vi "Authenticate without Token.vi"(5 "HTTP Method":T4, 6 "Body Parameters":T3[](array[typedef]), 7 "OAuth Credentials":T1={"Consumer Key"="", "Signature Method"=enum."HMAC-SHA1", "Token"="", "Version"="", "Token Secret"="", "Consumer Secret"=""}, 8 "error in (no error)":errorcluster, 9 "Header Parameters":T3[](array[typedef]), 10 "URL Parameters":T3[](array[typedef]), 11 "Base URL":string) -> (0 "error out":errorcluster, 1 "Header Value":string, 2 "Header Parameter":string, 3 "Full URL":string, 4 "Body":string)   [LabVIEW 2011, in "i3-oauth.lvlib"]
uses:
  i3-oauth.lvlib
  Controls/key-value-pairs.ctl
  Controls/HTTP Method.ctl
  Controls/OAuth Credentials.ctl
  Controls/Signature Method.ctl
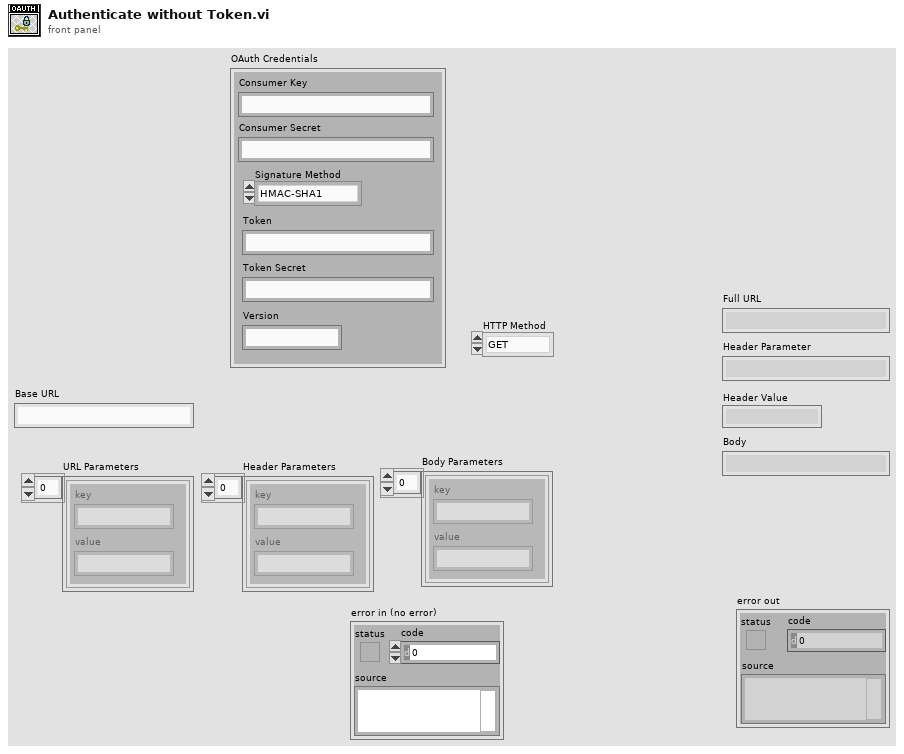
[diagram p1: front panel]
types:
  T1 = typedef "i3-oauth.lvlib/OAuth Credentials.ctl" = cluster{"Consumer Key":string, "Signature Method":T2, "Token":string, "Version":string, "Token Secret":string, "Consumer Secret":string}
  T2 = typedef "i3-oauth.lvlib/Signature Method.ctl" = enum16{"HMAC-MD5", "HMAC-SHA1", "HMAC-SHA224", "HMAC-SHA256", "HMAC-SHA384", "HMAC-SHA512"}
  T3 = typedef "i3-oauth.lvlib/key-value-pairs.ctl" = cluster{"key":string, "value":string}
  T4 = typedef "i3-oauth.lvlib/HTTP Method.ctl" = enum16{"GET", "POST", "PUT", "DELETE"}
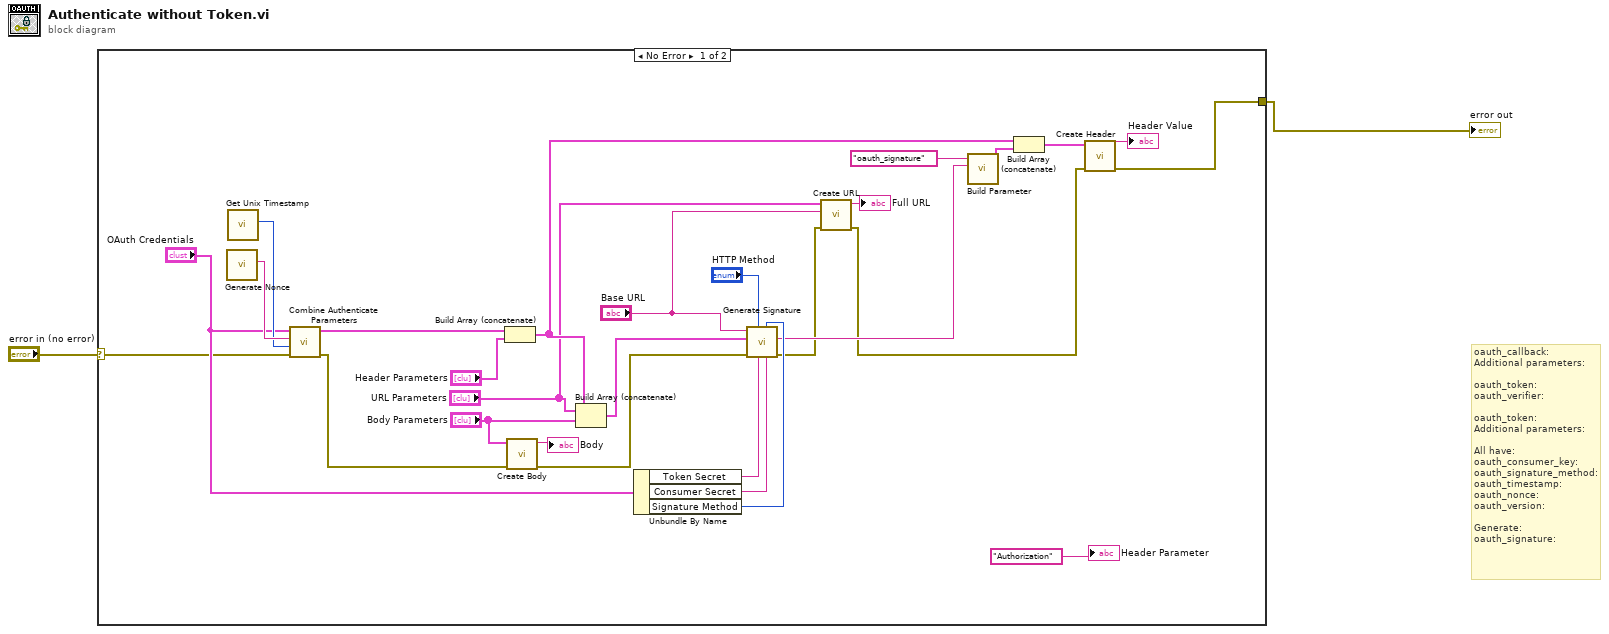
[diagram p0: block diagram]
diagram:
  # "oauth_callback:\nAdditional parameters:\n\noauth_token:\noauth_verifier:\n\noauth_token:\nAdditional parameters:\n\nAll have:\noauth_consumer_key:\noauth_signature_method:\noauth_timestamp:\noauth_nonce:\noauth_version:\n\nGenerate:\noauth_signature:"
  n1 = case shown="No Error" "error in (no error)" {
    selector: "error in (no error)" -> [w8 w31]
    tunnel: [w20 w31] -> w2
    frame No Error {
      n2 = call "Generate Nonce.vi"() -> ("nonce"=w27:string)  [unwired: 11 in]
      n3 = call "Get Unix Timestamp.vi"() -> ("Unix Timestamp"=w25:u64)  [unwired: 11 in]
      n4 = call "Combine Authenticate Parameters.vi"("error in (no error)"=w8, "Timestamp"=w25, "Nonce"=w27, "OAuth Credentials"="OAuth Credentials") -> ("error out"=w9:errorcluster, "Authentication Parameters"=w28:T3[])  [unwired: 6 in]
      n5 = Build Array (concatenate)(w28, "Header Parameters") -> (w18:T3[])
      n6 = call "Create Body.vi"("error in (no error)"=w9, "Body Parameters"="Body Parameters") -> ("error out"=w10:errorcluster, "Body"=→"Body":string)  [unwired: 8 in]
      n7 = Build Array (concatenate)(w18, "URL Parameters", "Body Parameters") -> (w26:T3[])
      n8 = Unbundle By Name("OAuth Credentials") -> ("Token Secret"=w24:string, "Consumer Secret"=w23:string, "Signature Method"=w19:T2)
      n9 = call "Generate Signature.vi"("consumer secret"=w23, "Signature Method"=w19, "token secret"=w24, "HTTP Method"="HTTP Method", "error in (no error)"=w10, "Parameters"=w26, "Base URL"="Base URL") -> ("error out"=w6:errorcluster, "Signature"=w11:string)  [unwired: 3 in]
      n10 = call "Create URL.vi"("error in (no error)"=w6, "Base URL"="Base URL", "URL Parameters"="URL Parameters") -> ("error out"=w5:errorcluster, "Full URL"=→"Full URL":string)  [unwired: 7 in]
      n11 = call "Build Parameter.vi"("Value"=w11, "Key"="oauth_signature" ("key")) -> ("Parameter Array"=w15:T3[])  [unwired: 9 in]
      n12 = Build Array (concatenate)(w18, w15) -> (w17:T3[])
      n13 = call "Create Header.vi"("error in (no error)"=w5, "Header Parameters"=w17) -> ("error out"=w20:errorcluster, "Header"=→"Header Value":string)  [unwired: 8 in]
      "Header Parameter" <- "Authorization"
    }
    frame Error {
    }
  }
  "error out" <- w2
